vi "Cal BC (Numeric).vi"(8 "error in (no error)":errorcluster, 10 "BC in":variant, 11 "Domain_Steady_2D_Polygon in":refnum<class "NI_Domain_Steady_2D_Polygon.lvclass">) -> (0 "error out":errorcluster, 2 "BC out":variant, 3 "Domain_Steady_2D_Polygon out":refnum<class "NI_Domain_Steady_2D_Polygon.lvclass">)   [LabVIEW 2020, in "NI_PDE.lvlib" / "NI_Domain_Steady_2D_Polygon.lvclass"]
uses:
  <vilib>/gmath/pde.llb/DomainClass/Domain_Steady_2D_Polygon/NI_Domain_Steady_2D_Polygon.lvclass
  <vilib>/gmath/pde.llb/BCClass/BC_Steady_2D_Numeric/BC Data.ctl
  <vilib>/gmath/pde.llb/Common/PDE_BC Type.ctl
  <vilib>/gmath/pde.llb/Common/PDE_BC Position 2D.ctl
  <vilib>/gmath/pde.llb/DomainClass/Domain_Steady_2D_Polygon/NI_Domain_Steady_2D_Polygon.lvclass/NI_Domain_Steady_2D_Polygon.ctl
  <vilib>/gmath/NI_PDE.lvlib
  <vilib>/gmath/pde.llb/BCClass/BC_Steady_2D_Numeric/NI_BC_Steady_2D_Numeric.lvclass
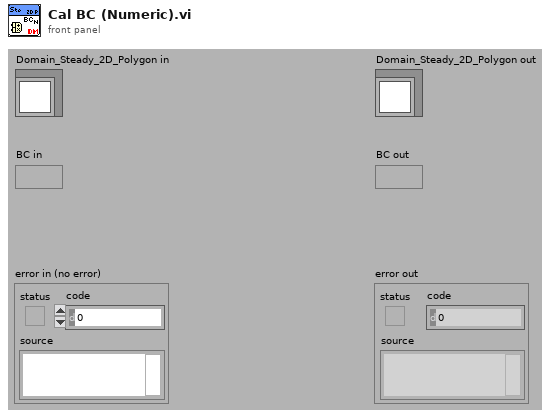
[diagram p1: front panel]
types:
  T1 = typedef "NI_PDE.lvlib/NI_BC_Steady_2D_Numeric.lvclass/BC Data.ctl" = cluster{"type":T2, "position":T3, "G":dbl[]}
  T2 = typedef "NI_PDE.lvlib/PDE_BC Type.ctl" = i32
  T3 = typedef "NI_PDE.lvlib/PDE_BC Position 2D.ctl" = i32
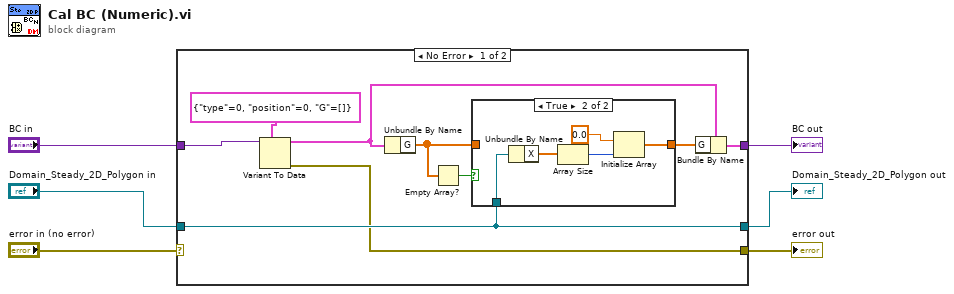
[diagram p0: block diagram]
diagram:
  n1 = case shown="No Error" "error in (no error)" {
    selector: "error in (no error)" -> [_ w24]
    tunnel: "Domain_Steady_2D_Polygon in" -> [w8 w23]
    tunnel: [w8 w23] -> w6
    tunnel: [w7 w24] -> w5
    tunnel: [w13 w22] -> w2
    tunnel: "BC in" -> [w14 w22]
    frame No Error {
      n2 = Variant To Data(type=T1 {"type"=0, "position"=0, "G"=[]} ("BC data"), Variant=w14) -> (data=w10:T1, error out=w7:errorcluster)  [unwired: 1 in]
      n3 = Unbundle By Name(w10) -> ("G"=w11:dbl[])
      n4 = Empty Array?(array=w11) -> (empty?=w12:bool)
      n5 = case shown="True" w12 {
        tunnel: w11 -> [w16 _]
        tunnel: [w16 w21] -> w9
        tunnel: w8 -> [_ w18]
        frame False {
        }
        frame True {
          n6 = Unbundle By Name(w18) -> ("X"=w17:dbl[])
          n7 = Array Size(array=w17) -> (size(s)=w19:i32)
          n8 = Initialize Array(0.0 ("element"), w19) -> (w21:dbl[])
        }
      }
      n9 = Bundle By Name(cluster=w10, "G"=w9) -> (w13:T1)
    }
    frame Error {
    }
  }
  "Domain_Steady_2D_Polygon out" <- w6
  "error out" <- w5
  "BC out" <- w2
